vi "SaveXferFnData.vi"(4 "XferFn":string[][](array[string]), 5 "ColumnTitle2":string="MyNameHere", 6 "ColumnTile1":string="MyNameHere", 7 "Inst (file) name":string="MyNameHere") -> (2 "Path name Out":path)   [LabVIEW 2020]
uses:
  Globals/Meas_global.vi
  Globals/Plug_in_data_global.vi
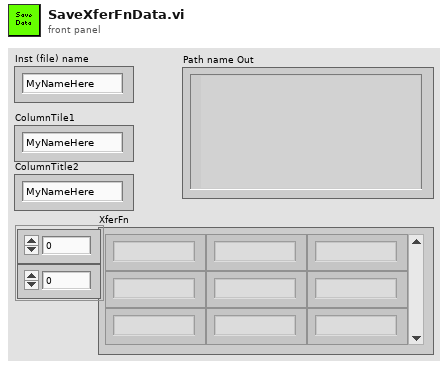
[diagram p1: front panel]
types:
  T1 = typedef "Post_Process.ctl" = enum16{"Take New Data", "Post Process Raw Data File"}
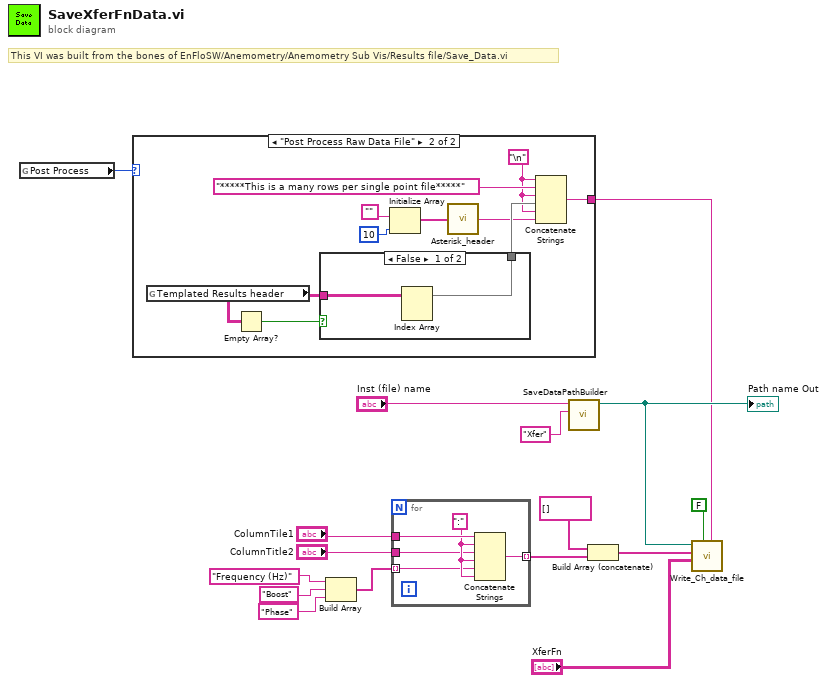
[diagram p0: block diagram]
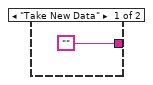
[diagram p2: hidden frame]
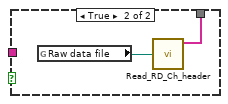
[diagram p3: hidden frame]
diagram:
  # "This VI was built from the bones of EnFloSW/Anemometry/Anemometry Sub Vis/Results file/Save_Data.vi"
  n1 = global read "Meas_global.vi" "Post Process"() -> (w16:T1)
  n2 = case shown="\"Post Process Raw Data File\"" w16 {
    tunnel: ["" w18] -> w6
    frame "Take New Data" {
    }
    frame "Post Process Raw Data File" {
      w19 = "\n"
      n3 = global read "Plug_in_data_global.vi" "Templated Results header"() -> (w24:string[][])
      n4 = Empty Array?(array=w24) -> (empty?=w26:bool)
      n5 = case shown="False" w26 {
        tunnel: [w28 w30] -> w25
        tunnel: w24 -> [w29 _]
        frame False {
          n6 = Index Array(array=w29) -> (element=w28:string[])  [unwired: 2 in]
        }
        frame True {
          n7 = global read "Meas_global.vi" "Raw data file"() -> (w31:path)
          n8 = call "Read_RD_Ch_header.vi"("Raw data file"=w31) -> ("Ch Name Out"=w30:string[])  [unwired: 3 out]
        }
      }
      n9 = Initialize Array("", 10) -> (w23:string[])
      n10 = call "Asterisk_header.vi"("Channel names"=w23) -> ("Header string"=w20:string)
      n11 = Concatenate Strings(w19, "*****This is a many rows per single point file*****", w19, w25, w19, w20) -> (w18:string)
    }
  }
  n12 = Build Array("Frequency (Hz)", "Boost", "Phase") -> (w11:string[])
  n13 = for {
    tunnel: "ColumnTile1" -> [w36]
    tunnel: "ColumnTitle2" -> [w34]
    tunnel: [w33] -> w12 mode=indexing
    tunnel: w11 -> [w32] mode=indexing
    w35 = ":" ("string")
    n14 = Concatenate Strings(w36, w35, w34, w35, w32, w35) -> (w33:string)
  }
  n15 = call "SaveDataPathBuilder.vi"("DataTypeSuffix"="Xfer", "Inst name"="Inst (file) name") -> ("Path name Out"=w13:path)  [unwired: 9 in]
  "Path name Out" <- w13
  n16 = Build Array (concatenate)(string[] [], w12) -> (w14:string[])
  n17 = call "Write_Ch_data_file.vi"("Header string"=w6, "exists?"=FALSE, "Channel Values"="XferFn", "Channel names"=w14, "Filename"=w13) -> ()  [unwired: 2 in, 5 out]
